vi "Konzentration aus Komponente ermitteln.vi"(10 "Index":i32, 11 "Gasflasche":u16) -> (3 "Konzentration IST":dbl)   [LabVIEW 2020, in "System Einstellungen V2.lvlib"]
uses:
  System Einstellungen V2.lvlib
  Aktion FGV Gasbottledefinition.ctl
  FT-IR/FGV FT-IR Gasliste Aktionen.ctl
  FT-IR/FT-IR.lvlib
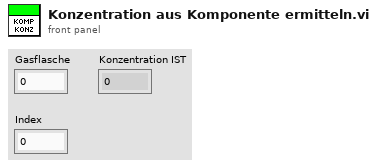
[diagram p1: front panel]
types:
  T1 = typedef "FT-IR.lvlib/FGV FT-IR Gasliste Aktionen.ctl" = enum16{"lesen", "Gasliste FT-IR", "Gasliste ausgelesen", "laden", "speichern", "löschen"}
  T2 = typedef "System Einstellungen V2.lvlib/Aktion FGV Gasbottledefinition.ctl" = enum16{"lesen", "schreiben", "löschen", "laden", "speichern", "exportieren", "importieren"}
  T3 = typedef "System Einstellungen V2.lvlib/Gasflasche gesamt.ctl" = cluster{"Gasflasche":T4, "Trägergas":T5, "Komponenten":T6[]}
  T4 = typedef "System Einstellungen V2.lvlib/Gasflasche.ctl" = cluster{"Gasname für die Auswahl":string, "Chargennummer":string, "Ablaufdatum":timestamp}
  T5 = typedef "System Einstellungen V2.lvlib/Traegergas.ctl" = string
  T6 = typedef "System Einstellungen V2.lvlib/Gasflaschenkomponente.ctl" = cluster{"Gasauswahl":string, "Konzentration IST":dbl, "Einheit":string, "Genauigkeit":dbl}
  T7 = typedef "String - Ausgabefeld.ctl" = string
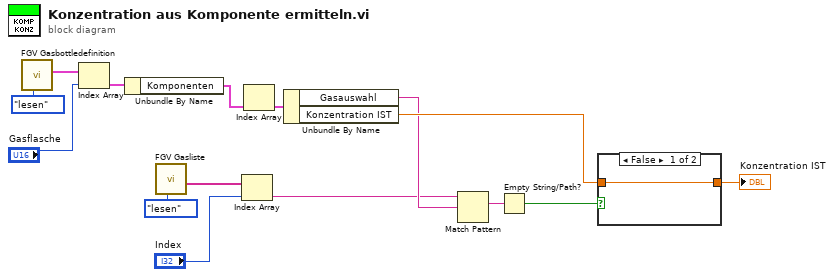
[diagram p0: block diagram]
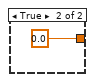
[diagram p2: hidden frame]
diagram:
  n1 = call "FGV Gasbottledefinition.vi"("Aktion"=Aktion_FGV_Gasbottledefinition."lesen") -> ("Gasflaschen Liste gesamt"=w15:T3[])  [unwired: 8 in, 2 out]
  n2 = Index Array(array=w15, index="Gasflasche") -> (element=w14:T3)
  n3 = Unbundle By Name(w14) -> ("Komponenten"=w12:T6[])
  n4 = call "FGV Gasliste.vi"("Aktionen"=FGV_FT-IR_Gasliste_Aktionen."lesen") -> ("Aktuelle Gasliste gesamt"=w8:T7[])  [unwired: 8 in, 2 out]
  n5 = Index Array(array=w8, index="Index") -> (element=w3:T7)
  n6 = Index Array(array=w12) -> (element=w13:T6)  [unwired: 1 in]
  n7 = Unbundle By Name(w13) -> ("Gasauswahl"=w4:string, "Konzentration IST"=w6:dbl)
  n8 = Match Pattern(string=w3, regular expression=w4) -> (match substring=w2:T7)  [unwired: 1 in, 3 out]
  n9 = Empty String/Path?(string/path=w2) -> (empty?=w1:bool)
  n10 = case shown="False" w1 {
    tunnel: w6 -> [w16 _]
    tunnel: [w16 0.0 ("Konzentration IST")] -> w5
    frame False {
    }
    frame True {
    }
  }
  "Konzentration IST" <- w5
